vi "Find Memory Address.vi"(4 "load data":T1={"max address"=0.0, "memory"="Digital Pattern Gen Memory 0"}, 10 ">=edge 1":bool, 11 "state data in":T2) -> (3 "state data out":T2)   [LabVIEW 2013, in "Engine Simulation Toolkit.lvlib" / "Digital Pattern Generation.lvlib"]
uses:
  Digital Pattern Generation.lvlib
  state data.ctl
  Load Data.ctl
  Engine Simulation Toolkit.lvlib
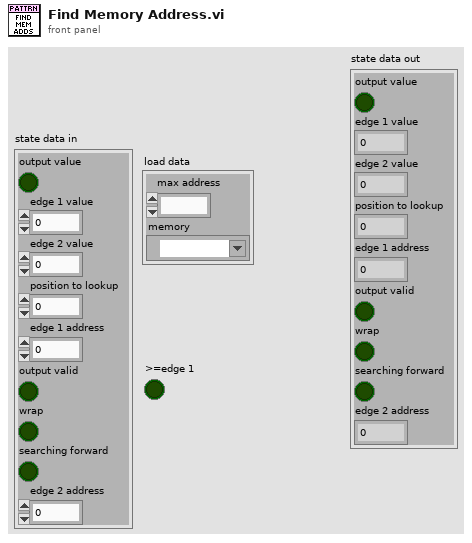
[diagram p1: front panel]
types:
  T1 = typedef "Engine Simulation Toolkit.lvlib/Digital Pattern Generation.lvlib/Load Data.ctl" = cluster{"max address":fxp<+,11,11>, "memory":refnum<k21>}
  T2 = typedef "Engine Simulation Toolkit.lvlib/Digital Pattern Generation.lvlib/state data.ctl" = cluster{"output value":bool, "edge 1 value":u16, "edge 2 value":u16, "position to lookup":u16, "edge 1 address":fxp<+,11,11>, "output valid":bool, "wrap":bool, "searching forward":bool, "edge 2 address":fxp<+,11,11>}
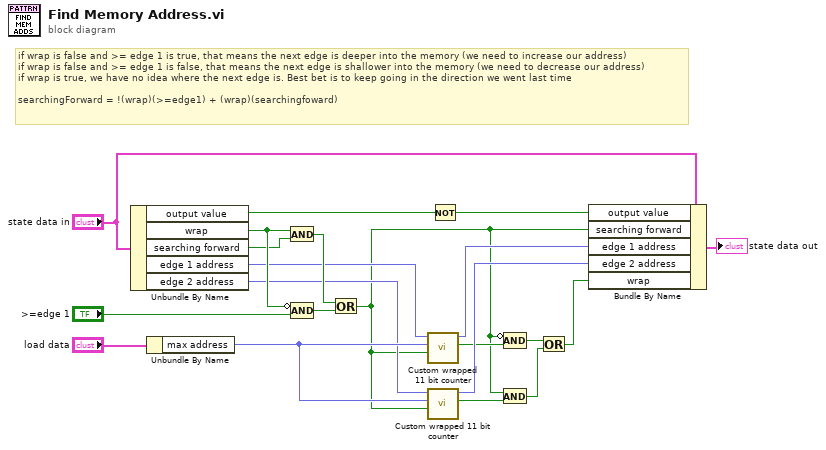
[diagram p0: block diagram]
diagram:
  # "if wrap is false and >= edge 1 is true, that means the next edge is deeper into the memory (we need to increase our address)\nif wrap is false and >= edge 1 is false, that means the next edge is shallower into the memory (we need to decrease our address)\nif wrap is true, we have no idea where the next edge is. Best bet is to keep going in the direction we went last time\n\nsearchingForward = !(wrap)(>=edge1) + (wrap)(searchingfoward)"
  n1 = Unbundle By Name("state data in") -> ("output value"=w13:bool, "wrap"=w16:bool, "searching forward"=w14:bool, "edge 1 address"=w10:fxp<+,11,11>, "edge 2 address"=w9:fxp<+,11,11>)
  n2 = Unbundle By Name("load data") -> ("max address"=w11:fxp<+,11,11>)
  n3 = And(x=w16, y=w14) -> (x .and. y?=w15:bool)
  n4 = Compound Arithmetic op=AND(invert w16, ">=edge 1") -> (w17:bool)
  n5 = Or(x=w15, y=w17) -> (x .or. y?=w3:bool)
  n6 = call "Custom wrapped 11 bit counter.vi"("increment or decrement (decrement)"=w3, "max value"=w11, "value"=w10) -> ("wrapped"=w4:bool, "new value"=w8:fxp<+,11,11>)  [unwired: 7 in]
  n7 = call "Custom wrapped 11 bit counter.vi"("increment or decrement (decrement)"=w3, "max value"=w11, "value"=w9) -> ("wrapped"=w2:bool, "new value"=w7:fxp<+,11,11>)  [unwired: 7 in]
  n8 = Not(x=w13) -> (.not. x?=w12:bool)
  n9 = And(x=w3, y=w2) -> (x .and. y?=w5:bool)
  n10 = Compound Arithmetic op=AND(invert w3, w4) -> (w6:bool)
  n11 = Or(x=w6, y=w5) -> (x .or. y?=w1:bool)
  n12 = Bundle By Name(cluster="state data in", "output value"=w12, "searching forward"=w3, "edge 1 address"=w8, "edge 2 address"=w7, "wrap"=w1) -> (→"state data out":T2)
